vi "Scrub.vi"(8 "error in":errorcluster, 10 "Input String":string, 11 "Regex Scrubber in":refnum<class "Regex Scrubber with Numbered Replacement.lvclass">) -> (0 "error out":errorcluster, 2 "Scrubbed String":string, 3 "Regex Scrubber out":refnum<class "Regex Scrubber with Numbered Replacement.lvclass">)   [LabVIEW 2020, in "Approval Tests.lvlib" / "Regex Scrubber with Numbered Replacement.lvclass"]
uses:
  Regex Scrubber with Numbered Replacement.lvclass
  Regex Scrubber with Numbered Replacement.lvclass/Regex Scrubber with Numbered Replacement.ctl
  <vilib>/regexp/Match Regular Expression.xnode
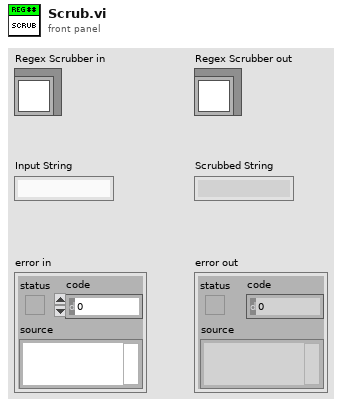
[diagram p1: front panel]
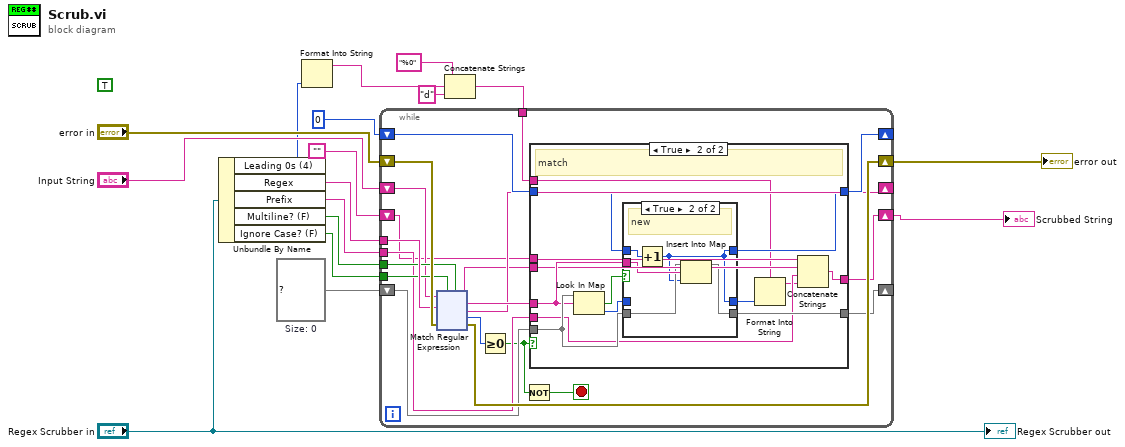
[diagram p0: block diagram]
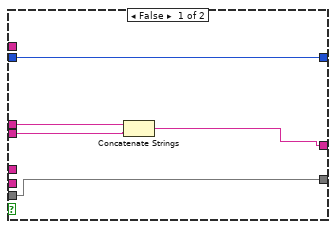
[diagram p2: hidden frame]
diagram:
  w8 = map{string, i32} {}  # Size: 0
  (unwired) TRUE ("replace all? (F)")
  n1 = Unbundle By Name("Regex Scrubber in") -> ("Leading 0s (4)"=w3:u32, "Regex"=w14:string, "Prefix"=w7:string, "Multiline? (F)"=w12:bool, "Ignore Case? (F)"=w13:bool)
  n2 = Format Into String(w3) -> (resulting string=w2:string)  [unwired: 3 in, 1 out]
  n3 = Concatenate Strings("%0" ("format string"), w2, "d" ("string")) -> (w4:string)
  n4 = while {
    shift-right: [w25] -> w6
    shift-left: "" -> [w19]
    tunnel: w14 -> [w35]
    tunnel: w13 -> [w34]
    tunnel: w12 -> [w33]
    shift-right: [w37] -> w16
    shift-left: "error in" -> [w36]
    shift-right: [w30] -> _
    shift-left: 0 -> [w31]
    shift-right: [w27] -> _
    shift-left: w8 -> [w28]
    tunnel: w7 -> [w26]
    shift-right: [w21] -> _
    shift-left: "Input String" -> [w32]
    tunnel: w4 -> [w18]
    stop <- w22 stop-if-true
    n5 = xnode "Match Regular Expression"("input string"=w32, "regular expression"=w35, "error in"=w36, "ignore case? (F)"=w34, "multiline? (F)"=w33) -> ("before match"=w20:string, "whole match"=w29:string, "after match"=w21:string, "offset past match"=w24:i32, "error out"=w37:errorcluster)  [unwired: 1 in]
    n6 = Greater Or Equal To 0?(x=w24) -> (x >= 0?=w23:bool)
    n7 = Not(x=w23) -> (.not. x?=w22:bool)
    n8 = case shown="True" w23 {
      tunnel: w31 -> [w41 w56]
      tunnel: [w41 w55] -> w30
      tunnel: w29 -> [_ w46]
      tunnel: w28 -> [w42 w54]
      tunnel: [w42 w53] -> w27
      tunnel: w26 -> [_ w50]
      tunnel: [w38 w47] -> w25
      tunnel: w20 -> [w40 w45]
      tunnel: w19 -> [w39 w44]
      tunnel: w18 -> [_ w43]
      frame False {
        n9 = Concatenate Strings(w39, w40) -> (w38:string)
      }
      frame True {
        # "match"
        n10 = Look In Map(map=w54, key=w46) -> (key not found?=w52:bool, value=w51:i32)  [unwired: 1 in]
        n11 = case shown="True" w52 {
          tunnel: w56 -> [w59 w64]
          tunnel: [w59 w60] -> w55
          tunnel: w46 -> [_ w63]
          tunnel: w54 -> [w58 w62]
          tunnel: [w58 w61] -> w53
          tunnel: w51 -> [w57 _]
          tunnel: [w57 w60] -> w49
          frame False {
            # "already there"
          }
          frame True {
            # "new"
            n12 = Increment(x=w64) -> (x+1=w60:i32)
            n13 = Insert Into Map(map in=w62, key=w63, value=w60) -> (map out=w61:map{string, i32})  [unwired: 2 out]
          }
        }
        n14 = Format Into String(format string=w43, w49) -> (resulting string=w48:string)  [unwired: 2 in, 1 out]
        n15 = Concatenate Strings(w44, w45, w50, w48) -> (w47:string)
      }
    }
  }
  "error out" <- w16
  "Scrubbed String" <- w6
  "Regex Scrubber out" <- "Regex Scrubber in"
